vi "Adjust_VI_Properties.vi"(6 "VI refnum in":refnum<vi>, 8 "error in (no error)":errorcluster, 9 "sourceInclusion":T3, 10 "properties in":T1[](array[typedef]), 11 "AB_DLL in":refnum<class "AB_DLL.lvclass">) -> (0 "error out":errorcluster, 1 "defaultSaveLevel":u32, 2 "properties out":T1[](array[typedef]), 3 "AB_DLL out":refnum<class "AB_DLL.lvclass">)   [LabVIEW 2020, in "AB_DLL.lvclass"]
uses:
  <vilib>/AppBuilder/AB_Classes/DLL/AB_DLL.lvclass
  <vilib>/AppBuilder/AB_Source_Properties.ctl
  <vilib>/AppBuilder/AB_Source_Property_Type.ctl
  <vilib>/AppBuilder/AB_Source_Inclusion.ctl
  <vilib>/AppBuilder/AB_Classes/Application/AB_Application.lvclass
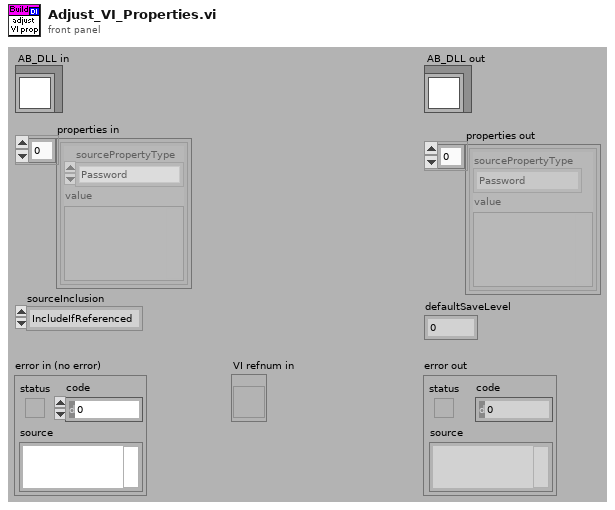
[diagram p1: front panel]
types:
  T1 = typedef "AB_Source_Properties.ctl" = cluster{"sourcePropertyType":T2, "value":variant}
  T2 = typedef "AB_Source_Property_Type.ctl" = enum16{"Remove block diagram", "Remove front panel", "Password", "Window has title bar", "Show menu bar", "Show vertical scroll bar", "Show horizontal scroll bar", "Show toolbar", "Show Abort button", "Show fp when called", "Window behavior", "Allow user to close window", "Window run-time position", "Run when opened", "Allow debugging", "Auto error handling", "Generate guard code", "Use stack variables", "Expression folding", "Integer only", "Inline subVI"}
  T3 = typedef "AB_Source_Inclusion.ctl" = enum16{"IncludeIfReferenced", "Include", "Exclude", "TopLevel"}
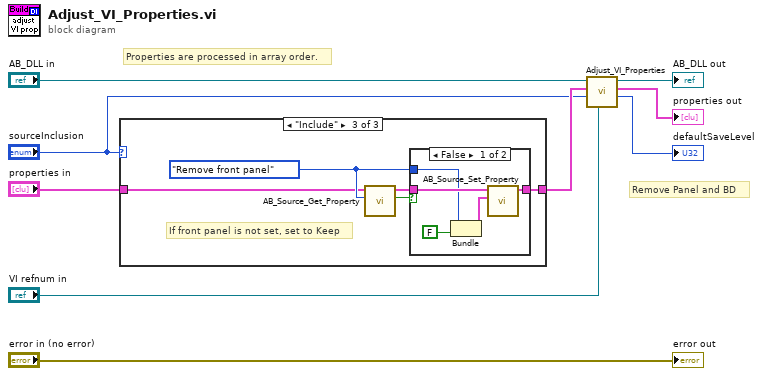
[diagram p0: block diagram]
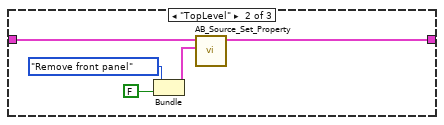
[diagram p3: hidden frame]
diagram:
  # "Remove Panel and BD"
  # "Properties are processed in array order."
  n1 = case shown="\"Include\"" "sourceInclusion" {
    tunnel: "properties in" -> [w10 w13 w17]
    tunnel: [w10 w11 w16] -> w5
    frame Default {
    }
    frame "TopLevel" {
      n2 = Bundle("sourcePropertyType"=AB_Source_Property_Type."Remove front panel", FALSE) -> (w12:cluster{"sourcePropertyType":T2, bool})  [unwired: 1 out]
      n3 = call <vilib>:"AB_Source_Set_Property.vi"("sourceProperty"=w12, "sourceProperties in"=w13) -> ("sourceProperties out"=w11:T1[])  [unwired: 1 in, 8 out]
    }
    frame "Include" {
      w20 = AB_Source_Property_Type."Remove front panel" ("sourcePropertyType")
      # "If front panel is not set, set to Keep"
      n4 = call <vilib>:"AB_Source_Get_Property.vi"("type"=w20, "sourceProperties in"=w17) -> ("found"=w18:bool, "sourceProperties out"=w19:T1[])  [unwired: 1 in, 7 out]
      n5 = case shown="False" w18 {
        tunnel: w19 -> [w25 w26]
        tunnel: [w24 w26] -> w16
        tunnel: w20 -> [w22 _]
        frame False {
          n6 = Bundle("sourcePropertyType"=w22, FALSE) -> (w21:cluster{"sourcePropertyType":T2, bool})  [unwired: 1 out]
          n7 = call <vilib>:"AB_Source_Set_Property.vi"("sourceProperty"=w21, "sourceProperties in"=w25) -> ("sourceProperties out"=w24:T1[])  [unwired: 1 in, 8 out]
        }
        frame True {
        }
      }
    }
  }
  n8 = call-parent "Adjust_VI_Properties.vi"("VI refnum in"="VI refnum in", "sourceInclusion"="sourceInclusion", "properties in"=w5, "AB_Application in"="AB_DLL in") -> ("defaultSaveLevel"=→"defaultSaveLevel":u32, "properties out"=→"properties out":T1[], "AB_Application out"=→"AB_DLL out":refnum<class "AB_DLL.lvclass">)  [unwired: 1 in, 4 out]
  "error out" <- "error in (no error)"
